vi "Wrap To World.vi"(11 "World Position":T1) -> (3 "World Position (Wrapped)":T1)   [LabVIEW 2018]
uses:
  LabSDL2/Source/Libraries/SDL2 Utility/Point (I32).ctl
  Math/Math.lvlib
  LabSDL2/Source/Libraries/SDL2 Utility/SDL2 Utility.lvlib
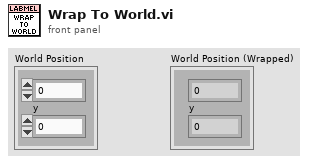
[diagram p1: front panel]
types:
  T1 = typedef "SDL2 Utility.lvlib/Point (I32).ctl" = cluster{"x":i32, "y":i32}
  T2 = typedef "Constants.ctl" = cluster{"Colours":cluster{"OK":u32, "Warning":u32, "Error":u32, "Red":u32, "Green":u32, "Blue":u32, "Yellow":u32}, "System":cluster{"Target Frames Second":dbl, "World Size":T1, "Window Size":T1, "Viewport Size":T1, "Sidebar Scaling":sgl, "Sidebar Width":i32, "SC2 Frame Rate [Seconds/Frame]":sgl}, "Game":cluster{"Maximum Asteroids":i32, "Max Energy":i32, "Max Crew":i32, "Maximum Stars":i32}}
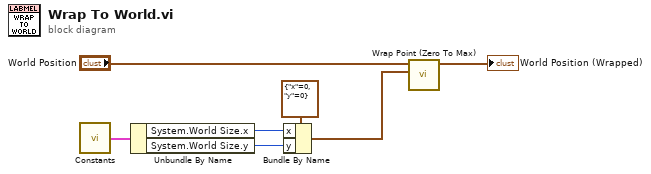
[diagram p0: block diagram]
diagram:
  n1 = call "Constants.vi"() -> ("Constants"=w6:T2)
  n2 = Unbundle By Name(w6) -> ("System.World Size.x"=w4:i32, "System.World Size.y"=w3:i32)
  n3 = Bundle By Name(cluster=T1 {"x"=0, "y"=0} ("World Position (Wrapped)"), "x"=w4, "y"=w3) -> (w2:T1)
  n4 = call "Wrap Point (Zero To Max).vi"("Max"=w2, "Point"="World Position") -> ("Point (Wrapped)"=→"World Position (Wrapped)":T1)  [unwired: 9 in]
